vi "camera mjpeg.vi"(11 "CameraDevRef":T1) -> ()   [LabVIEW 2013]
uses:
  <vilib>/Rock Robotics/WPI/Camera/WPI_CameraDevRef.ctl
  <vilib>/Rock Robotics/WPI/Camera/WPI_CameraSettings Operations.ctl
  typedefs/fg_typedef.ctl
  typedefs/Vision/vision enable.ctl
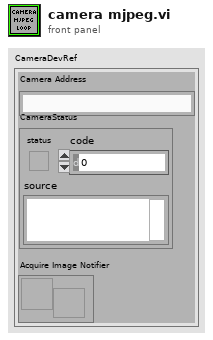
[diagram p1: front panel]
types:
  T1 = typedef "WPI_CameraDevRef.ctl" = cluster{"Camera Address":string, "CameraStatus":errorcluster, "Acquire Image Notifier":refnum<notifier>}
  T2 = typedef "WPI_CameraSettings Operations.ctl" = enum16{"Udate FPS", "Update Compression", "Update Size", "Update White Balance", "Update Brightness", "Update Sharpness", "Update Exposure", "Update Color Level", "Update Exp Priority", "Update Color Enable", "Update JPG", "Update MJPG", "Read and Clear", "Read", "Init"}
  T3 = typedef "vision enable.ctl" = enum16{"Enable", "Disable", "Stop"}
  T4 = typedef "fg_typedef.ctl" = enum16{"Get", "Set"}
  T5 = typedef "WPI_CameraSettings Control.ctl" = cluster{"FPS":i32, "Compression":i32, "Size":i32, "White Balance":i32, "Brightness":i32, "Sharpness":i32, "Exposure":i32, "Color Level":i32, "Exposure Priority":i32, "Color Enable":i32, "JPG Loop":i32, "MJPG Loop":i32}
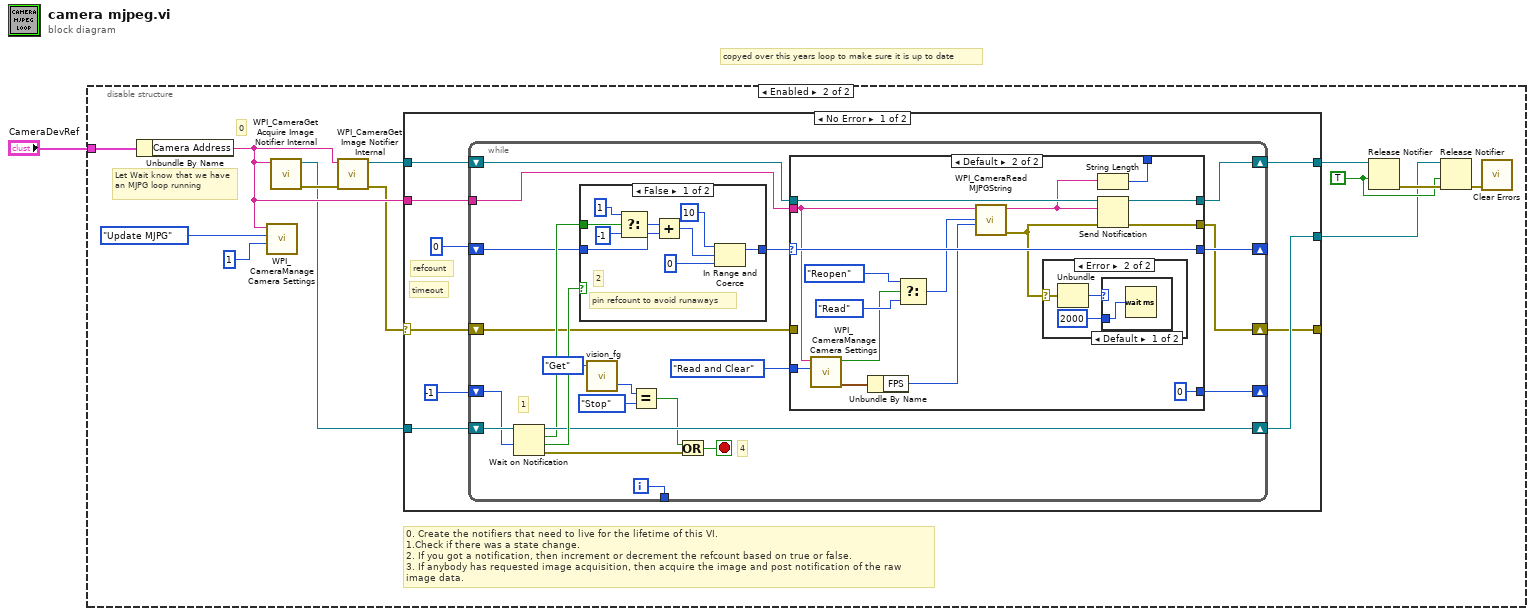
[diagram p0: block diagram]
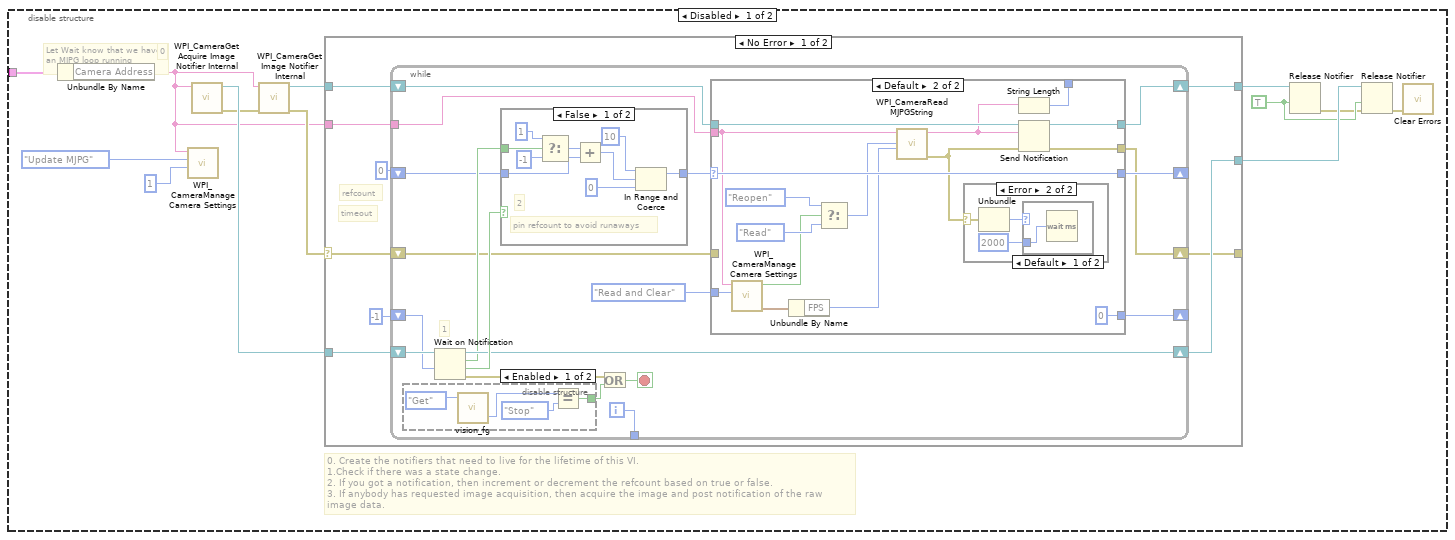
[diagram p2: hidden frame]
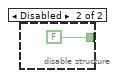
[diagram p3: hidden frame]
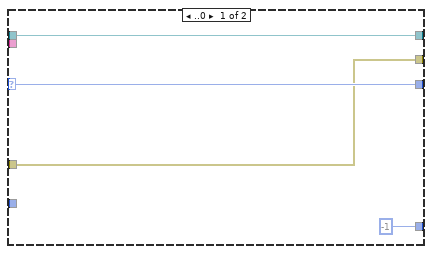
[diagram p4: hidden frame]
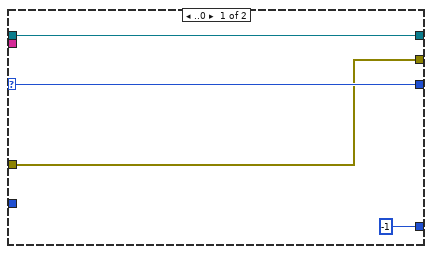
[diagram p9: hidden frame]
diagram:
  # "copyed over this years loop to make sure it is up to date"
  n1 = disable-structure shown="Enabled" {
    disable-tunnel: "CameraDevRef" -> [w10 w85]
    frame Disabled {
      w11 = TRUE ("force destroy? (F)")
      # "Let Wait know that we have\nan MJPG loop running"
      # "0"
      # "0. Create the notifiers that need to live for the lifetime of this VI. \n1.Check if there was a state change.\n2. If you got a notification, then increment or decrement the refcount based on true or false.\n3. If anybody has requested image acquisition, then acquire the image and post notification of the raw image data."
      n2 = Unbundle By Name(w10) -> ("Camera Address"=w2:string)
      n3 = call <vilib>:"WPI_CameraManage Camera Settings.vi"("Value"=1, "Operation"=WPI_CameraSettings_Operations."Update MJPG", "Camera IP"=w2) -> ()  [unwired: 7 in, 2 out]
      n4 = call <vilib>:"WPI_CameraGet Acquire Image Notifier Internal.vi"("Camera Address"=w2) -> ("error out"=w6:errorcluster, "Acquire Image Notifier"=w7:refnum<notifier>)  [unwired: 1 in, 8 out]
      n5 = call <vilib>:"WPI_CameraGet Image Notifier Internal.vi"("error in (no error)"=w6, "Camera Address"=w2) -> ("error out"=w9:errorcluster, "Image Notifier"=w12:refnum<notifier>)  [unwired: 8 out]
      n6 = case shown="No Error" w9 {
        selector: w9 -> [w16 w84]
        tunnel: w2 -> [w23 _]
        tunnel: w7 -> [w22 w82]
        tunnel: w12 -> [w20 w83]
        tunnel: [w18 w83] -> w14
        tunnel: [w17 w82] -> w13
        tunnel: [w15 w84] -> _
        frame No Error {
          # "timeout"
          # "refcount"
          n7 = while {
            shift-right: [w40] -> w17
            shift-left: w22 -> [w42]
            tunnel: w23 -> [w37]
            shift-right: [w30] -> _
            shift-left: 0 -> [w38]
            shift-right: [w35] -> w18
            shift-left: w20 -> [w36]
            shift-right: [w33] -> _
            shift-left: -1 -> [w34]
            shift-right: [w29] -> w15
            shift-left: w16 -> [w32]
            tunnel: [w27] -> _
            i -> [w27]
            stop <- w26 stop-if-true
            # "1"
            n8 = disable-structure shown="Enabled" {
              disable-tunnel: [w43 FALSE] -> w24
              frame Enabled {
                n9 = call "vision_fg.vi"("Menu"=fg_typedef."Get") -> ("State Out"=w45:T3)  [unwired: 2 in, 1 out]
                n10 = Equal?(x=w45, y=vision_enable."Stop") -> (x = y?=w43:bool)
              }
              frame Disabled {
              }
            }
            n11 = Wait on Notification(notifier=w42, timeout in ms (-1)=w34) -> (notifier out=w40:refnum<notifier>, notification=w39:bool, timed out?=w41:bool, error out=w25:errorcluster)  [unwired: 1 in, 1 out]
            n12 = case shown="False" w41 {
              tunnel: w39 -> [w80 _]
              tunnel: w38 -> [w76 w81]
              tunnel: [w72 w81] -> w31
              frame False {
                # "pin refcount to avoid runaways"
                # "2"
                n13 = Select(t=1, s=w80, f=-1) -> (s? t:f=w77:i32)
                n14 = Add(x=w77, y=w76) -> (x+y=w73:i32)
                n15 = In Range and Coerce(upper limit=10, x=w73, lower limit=0) -> (coerced(x)=w72:i32)  [unwired: 1 out]
              }
              frame True {
              }
            }
            n16 = Or(x=w25, y=w24) -> (x .or. y?=w26:bool)
            n17 = case shown="Default" w31 {
              selector: w31 -> [w50 w64]
              tunnel: w37 -> [_ w52]
              tunnel: w36 -> [w51 w67]
              tunnel: [w51 w66] -> w35
              tunnel: [-1 0] -> w33
              tunnel: w32 -> [w48 _]
              tunnel: [w50 w64] -> w30
              tunnel: [w48 w63] -> w29
              tunnel: [_ w57] -> _
              tunnel: WPI_CameraSettings_Operations."Read and Clear" ("Operation") -> [_ w53]
              frame ..0 {
              }
              frame Default {
                n18 = call <vilib>:"WPI_CameraManage Camera Settings.vi"("Operation"=w53, "Camera IP"=w52) -> ("Values"=w55:T5, "Changed"=w56:bool)  [unwired: 8 in]
                n19 = Unbundle By Name(w55) -> ("FPS"=w54:i32)
                n20 = Select(t=enum16{"Read", "Reopen", "Close"}."Reopen" ("Operation"), s=w56, f=enum16{"Read", "Reopen", "Close"}."Read" ("Operation")) -> (s? t:f=w59:enum16{"Read", "Reopen", "Close"})
                n21 = call <vilib>:"WPI_CameraRead MJPGString.vi"("fps"=w54, "Operation"=w59, "address"=w52) -> ("error out"=w62:errorcluster, "Raw Image Data"=w58:string)  [unwired: 7 in]
                n22 = case shown="Error" w62 {
                  selector: w62 -> [_ w70]
                  frame No Error {
                  }
                  frame Error {
                    n23 = Unbundle(w70) -> ("code"=w69:i32)  [unwired: 2 out]
                    n24 = case shown="Default" w69 {
                      tunnel: u32 2000 ("milliseconds to wait") -> [w71 _]
                      frame Default {
                        n25 = Wait (ms)(milliseconds to wait=w71) -> ()  [unwired: 1 out]
                      }
                      frame 56 {
                      }
                    }
                  }
                }
                n26 = String Length(string=w58) -> (length=w57:i32)
                n27 = Send Notification(notification=w58, notifier=w67, error in (no error)=w62) -> (notifier out=w66:refnum<notifier>, error out=w63:errorcluster)
              }
            }
          }
        }
        frame Error {
        }
      }
      n28 = Release Notifier(notifier=w14, force destroy? (F)=w11) -> (error out=w5:errorcluster)  [unwired: 1 in, 2 out]
      n29 = Release Notifier(notifier=w13, force destroy? (F)=w11, error in (no error)=w5) -> (error out=w8:errorcluster)  [unwired: 2 out]
      n30 = call <vilib>:"Clear Errors.vi"("error in (no error)"=w8) -> ()  [unwired: 7 out]
    }
    frame Enabled {
      w89 = TRUE ("force destroy? (F)")
      # "Let Wait know that we have\nan MJPG loop running"
      # "0"
      # "0. Create the notifiers that need to live for the lifetime of this VI. \n1.Check if there was a state change.\n2. If you got a notification, then increment or decrement the refcount based on true or false.\n3. If anybody has requested image acquisition, then acquire the image and post notification of the raw image data."
      n31 = Unbundle By Name(w85) -> ("Camera Address"=w97:string)
      n32 = call <vilib>:"WPI_CameraManage Camera Settings.vi"("Value"=1, "Operation"=WPI_CameraSettings_Operations."Update MJPG", "Camera IP"=w97) -> ()  [unwired: 7 in, 2 out]
      n33 = call <vilib>:"WPI_CameraGet Acquire Image Notifier Internal.vi"("Camera Address"=w97) -> ("error out"=w93:errorcluster, "Acquire Image Notifier"=w92:refnum<notifier>)  [unwired: 1 in, 8 out]
      n34 = call <vilib>:"WPI_CameraGet Image Notifier Internal.vi"("error in (no error)"=w93, "Camera Address"=w97) -> ("error out"=w90:errorcluster, "Image Notifier"=w88:refnum<notifier>)  [unwired: 8 out]
      n35 = case shown="No Error" w90 {
        selector: w90 -> [w99 w165]
        tunnel: w97 -> [w106 _]
        tunnel: w92 -> [w105 w163]
        tunnel: w88 -> [w103 w164]
        tunnel: [w101 w164] -> w86
        tunnel: [w100 w163] -> w87
        tunnel: [w98 w165] -> _
        frame No Error {
          # "timeout"
          # "refcount"
          n36 = while {
            shift-right: [w126] -> w100
            shift-left: w105 -> [w128]
            tunnel: w106 -> [w123]
            shift-right: [w115] -> _
            shift-left: 0 -> [w124]
            shift-right: [w121] -> w101
            shift-left: w103 -> [w122]
            shift-right: [w119] -> _
            shift-left: -1 -> [w120]
            shift-right: [w114] -> w98
            shift-left: w99 -> [w117]
            tunnel: [w112] -> _
            i -> [w112]
            stop <- w108 stop-if-true
            # "4"
            # "1"
            n37 = Wait on Notification(notifier=w128, timeout in ms (-1)=w120) -> (notifier out=w126:refnum<notifier>, notification=w125:bool, timed out?=w127:bool, error out=w118:errorcluster)  [unwired: 1 in, 1 out]
            n38 = case shown="False" w127 {
              tunnel: w125 -> [w161 _]
              tunnel: w124 -> [w157 w162]
              tunnel: [w153 w162] -> w116
              frame False {
                # "pin refcount to avoid runaways"
                # "2"
                n39 = Select(t=1, s=w161, f=-1) -> (s? t:f=w158:i32)
                n40 = Add(x=w158, y=w157) -> (x+y=w154:i32)
                n41 = In Range and Coerce(upper limit=10, x=w154, lower limit=0) -> (coerced(x)=w153:i32)  [unwired: 1 out]
              }
              frame True {
              }
            }
            n42 = call "vision_fg.vi"("Menu"=fg_typedef."Get") -> ("State Out"=w110:T3)  [unwired: 2 in, 1 out]
            n43 = Equal?(x=w110, y=vision_enable."Stop") -> (x = y?=w107:bool)
            n44 = Or(x=w107, y=w118) -> (x .or. y?=w108:bool)
            n45 = case shown="Default" w116 {
              selector: w116 -> [w131 w145]
              tunnel: w123 -> [_ w133]
              tunnel: w122 -> [w132 w148]
              tunnel: [w132 w147] -> w121
              tunnel: [-1 0] -> w119
              tunnel: w117 -> [w129 _]
              tunnel: [w131 w145] -> w115
              tunnel: [w129 w144] -> w114
              tunnel: [_ w138] -> _
              tunnel: WPI_CameraSettings_Operations."Read and Clear" ("Operation") -> [_ w134]
              frame ..0 {
              }
              frame Default {
                n46 = call <vilib>:"WPI_CameraManage Camera Settings.vi"("Operation"=w134, "Camera IP"=w133) -> ("Values"=w136:T5, "Changed"=w137:bool)  [unwired: 8 in]
                n47 = Unbundle By Name(w136) -> ("FPS"=w135:i32)
                n48 = Select(t=enum16{"Read", "Reopen", "Close"}."Reopen" ("Operation"), s=w137, f=enum16{"Read", "Reopen", "Close"}."Read" ("Operation")) -> (s? t:f=w140:enum16{"Read", "Reopen", "Close"})
                n49 = call <vilib>:"WPI_CameraRead MJPGString.vi"("fps"=w135, "Operation"=w140, "address"=w133) -> ("error out"=w143:errorcluster, "Raw Image Data"=w139:string)  [unwired: 7 in]
                n50 = case shown="Error" w143 {
                  selector: w143 -> [_ w151]
                  frame No Error {
                  }
                  frame Error {
                    n51 = Unbundle(w151) -> ("code"=w150:i32)  [unwired: 2 out]
                    n52 = case shown="Default" w150 {
                      tunnel: u32 2000 ("milliseconds to wait") -> [w152 _]
                      frame Default {
                        n53 = Wait (ms)(milliseconds to wait=w152) -> ()  [unwired: 1 out]
                      }
                      frame 56 {
                      }
                    }
                  }
                }
                n54 = String Length(string=w139) -> (length=w138:i32)
                n55 = Send Notification(notification=w139, notifier=w148, error in (no error)=w143) -> (notifier out=w147:refnum<notifier>, error out=w144:errorcluster)
              }
            }
          }
        }
        frame Error {
        }
      }
      n56 = Release Notifier(notifier=w86, force destroy? (F)=w89) -> (error out=w94:errorcluster)  [unwired: 1 in, 2 out]
      n57 = Release Notifier(notifier=w87, force destroy? (F)=w89, error in (no error)=w94) -> (error out=w91:errorcluster)  [unwired: 2 out]
      n58 = call <vilib>:"Clear Errors.vi"("error in (no error)"=w91) -> ()  [unwired: 7 out]
    }
  }
